vi "通讯test.vi"() -> ()   [LabVIEW 2012]
uses:
  <vilib>/Instr/_visa.llb/VISA Configure Serial Port (Instr).vi
panel:
  in  "文本输入":string
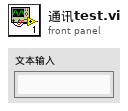
[diagram p1: front panel]
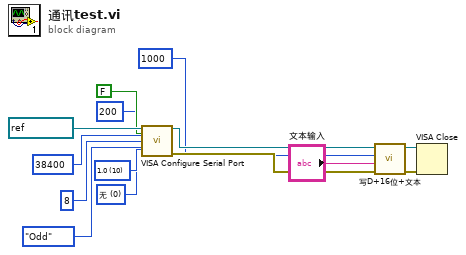
[diagram p0: block diagram]
diagram:
  w8 = u16 0 items=["无", "XON/XOFF", "RTS/CTS", "XON/XOFF & RTS/CTS", "DTR/DSR", "XON/XOFF & DTR/DSR"] ("flow control (0:none)")
  w9 = u16 10 items=["1.0"=10, "1.5"=15, "2.0"=20] ("stop bits (10: 1 bit)")
  n1 = call-poly "VISA Configure Serial Port"("VISA resource name"=refnum<visa-resource-name> "COM3", "timeout (10sec)"=u32 200, "Enable Termination\nChar (T)"=FALSE ("Enable Termination\nChar (T)"), "baud rate (9600)"=u32 38400, "data bits (8)"=u16 8, "parity (0:none)"=enum16{"None", "Odd", "Even", "Mark", "Space"}."Odd", "stop bits (10: 1 bit)"=w9, "flow control (0:none)"=w8) -> ("VISA resource name out"=w6:refnum<visa-resource-name>, "error out"=w5:errorcluster)  [unwired: 6 in]
  n2 = call "写D+16位+文本.vi"("error out"=w5, "文本输入"="文本输入", "输入地址D"=1000 ("读取D地址"), "VISA resource name out"=w6) -> ("error out 2"=w3:errorcluster, "VISA resource name out 2"=w4:refnum<visa-resource-name>)  [unwired: 3 in, 3 out]
  n3 = VISA Close(VISA resource name=w4, error in (no error)=w3) -> ()  [unwired: 1 out]
